vi "Helper-SubPanel.vi"() -> ()   [LabVIEW 2016, in "test_ValueSignal.lvlib"]
uses:
  test_ValueSignal.lvlib
  SubVi/SubPanelVI2.vi
  SubVi/SubPanelVI1.vi
panel:
  in  "Load SP1":bool
  in  "Remove":bool
  out "error out":errorcluster
  in  "stop":bool
  in  "Load SP2":bool
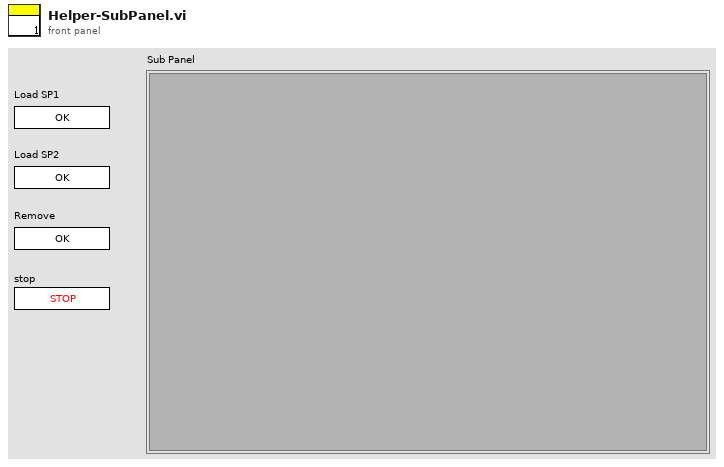
[diagram p1: front panel]
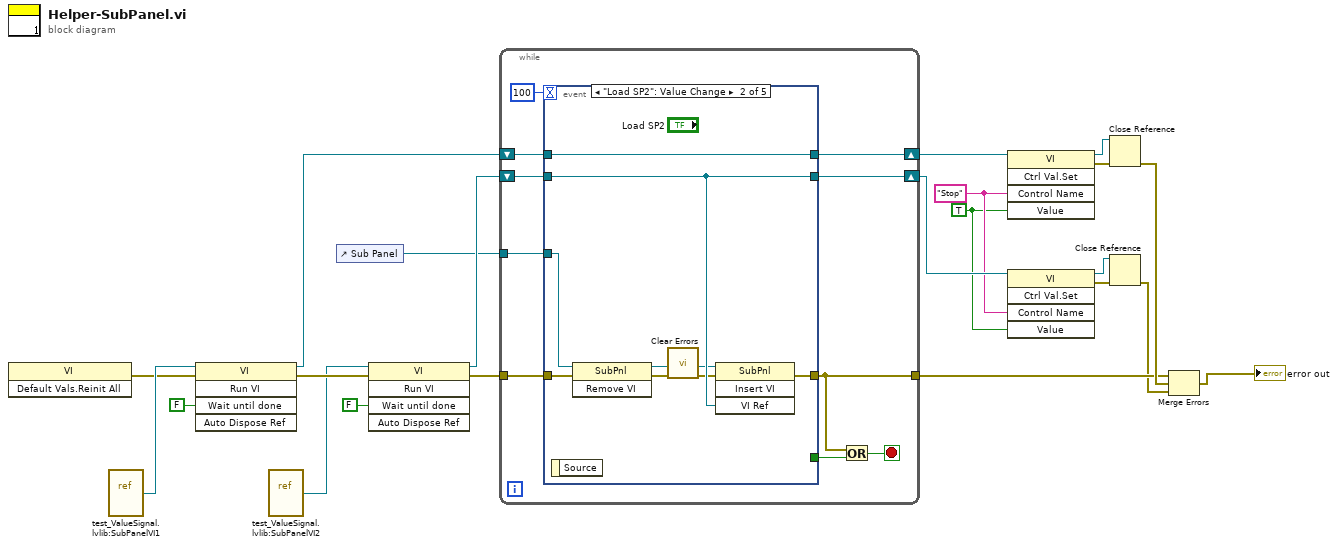
[diagram p0: block diagram]
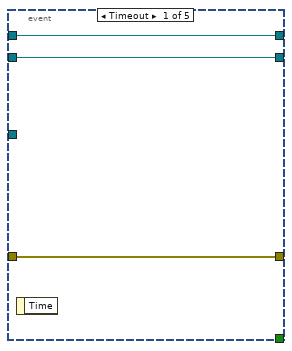
[diagram p2: hidden frame]
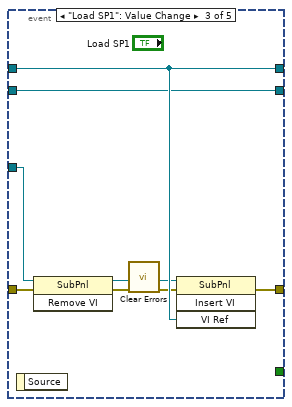
[diagram p3: hidden frame]
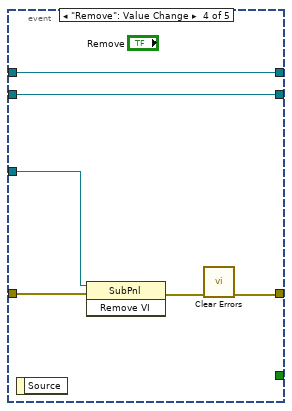
[diagram p4: hidden frame]
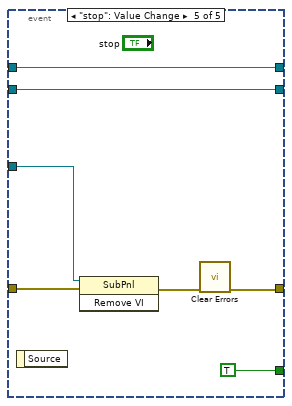
[diagram p5: hidden frame]
diagram:
  w3 = TRUE
  w4 = "Stop" ("Control Name")
  n1 = invoke class="VI" method="Default Vals.Reinit All"() -> (error out=w2:errorcluster)  [unwired: 3 in, 2 out]
  n2 = vi-ref "test_ValueSignal.lvlib:SubPanelVI1.vi"() -> (w15:refnum<vi>)
  n3 = invoke class="VI" method="Run VI"(reference=w15, error in=w2, "Wait until done"=FALSE ("Wait Until Done")) -> (reference out=w19:refnum<vi>, error out=w17:errorcluster)  [unwired: 2 in, 3 out]
  n4 = vi-ref "test_ValueSignal.lvlib:SubPanelVI2.vi"() -> (w16:refnum<vi>)
  n5 = control-ref of="Sub Panel"() -> (w1:refnum<vi>)
  n6 = invoke class="VI" method="Run VI"(reference=w16, error in=w17, "Wait until done"=FALSE ("Wait Until Done")) -> (reference out=w22:refnum<vi>, error out=w14:errorcluster)  [unwired: 2 in, 3 out]
  n7 = while {
    tunnel: w14 -> [w31]
    tunnel: [w26] -> w6
    shift-right: [w28] -> w10
    shift-left: w19 -> [w29]
    shift-right: [w27] -> w11
    shift-left: w22 -> [w30]
    tunnel: w1 -> [w23]
    stop <- w24 stop-if-true
    n8 = event shown="[1] \"Load SP2\": Value Change" {
      selector: _ -> [_ _ _ _ _]
      dyn-events: _ -> [_ _ _ _ _]
      timeout: 100 -> [_ _ _ _ _]
      tunnel: w31 -> [w35 w41 w50 w57 w64]
      tunnel: [w35 w42 w51 w52 w58] -> w26
      tunnel: w30 -> [w33 w43 w47 w54 w60]
      tunnel: w29 -> [w34 w39 w48 w55 w61]
      tunnel: [_ _ _ _ TRUE ("stop")] -> w25
      tunnel: [w34 w39 w48 w55 w61] -> w28
      tunnel: [w33 w43 w47 w54 w60] -> w27
      tunnel: w23 -> [_ w38 w46 w53 w59]
      event Timeout {
        n9 = event-data() -> ()  [unwired: 1 in, 1 out]
      }
      event "Load SP2": Value Change {
        n10 = event-data() -> ()  [unwired: 1 in, 1 out]
        n11 = invoke on="Invoke Node" class="SubPnl" method="Remove VI"(reference=w38, error in=w41) -> (reference out=w37:refnum<vi>, error out=w40:errorcluster)  [unwired: 1 in, 1 out]
        n12 = call <vilib>:"Clear Errors.vi"("error in (no error)"=w40) -> ("error out"=w36:errorcluster)  [unwired: 5 in, 1 out]
        n13 = invoke on="Invoke Node" class="SubPnl" method="Insert VI"(reference=w37, error in=w36, "VI Ref"=w43) -> (error out=w42:errorcluster)  [unwired: 1 in, 3 out]
      }
      event "Load SP1": Value Change {
        n14 = event-data() -> ()  [unwired: 1 in, 1 out]
        n15 = invoke on="Invoke Node" class="SubPnl" method="Remove VI"(reference=w46, error in=w50) -> (reference out=w45:refnum<vi>, error out=w49:errorcluster)  [unwired: 1 in, 1 out]
        n16 = call <vilib>:"Clear Errors.vi"("error in (no error)"=w49) -> ("error out"=w44:errorcluster)  [unwired: 5 in, 1 out]
        n17 = invoke on="Invoke Node" class="SubPnl" method="Insert VI"(reference=w45, error in=w44, "VI Ref"=w48) -> (error out=w51:errorcluster)  [unwired: 1 in, 3 out]
      }
      event "Remove": Value Change {
        n18 = event-data() -> ()  [unwired: 1 in, 1 out]
        n19 = invoke on="Invoke Node" class="SubPnl" method="Remove VI"(reference=w53, error in=w57) -> (error out=w56:errorcluster)  [unwired: 1 in, 2 out]
        n20 = call <vilib>:"Clear Errors.vi"("error in (no error)"=w56) -> ("error out"=w52:errorcluster)  [unwired: 5 in, 1 out]
      }
      event "stop": Value Change {
        n21 = event-data() -> ()  [unwired: 1 in, 1 out]
        n22 = invoke on="Invoke Node" class="SubPnl" method="Remove VI"(reference=w59, error in=w64) -> (error out=w63:errorcluster)  [unwired: 1 in, 2 out]
        n23 = call <vilib>:"Clear Errors.vi"("error in (no error)"=w63) -> ("error out"=w58:errorcluster)  [unwired: 5 in, 1 out]
      }
    }
    n24 = Or(x=w26, y=w25) -> (x .or. y?=w24:bool)
  }
  n25 = invoke class="VI" method="Ctrl Val.Set"(reference=w10, "Control Name"=w4, "Value"=w3) -> (reference out=w9:refnum<vi>, error out=w8:errorcluster)  [unwired: 2 in, 3 out]
  n26 = invoke class="VI" method="Ctrl Val.Set"(reference=w11, "Control Name"=w4, "Value"=w3) -> (reference out=w12:refnum<vi>, error out=w13:errorcluster)  [unwired: 2 in, 3 out]
  n27 = Close Reference(reference=w9, error in (no error)=w8) -> (error out=w18:errorcluster)
  n28 = Close Reference(reference=w12, error in (no error)=w13) -> (error out=w5:errorcluster)
  n29 = Merge Errors(w6, w18, w5) -> (→"error out":errorcluster)
